vi "Generate Cartesian Trajectory.vi"   [LabVIEW 2017, in "NI_Kinematics.lvlib"]
doc: "Generates a smooth trajectory of end effector positions between two points in Cartesian space. Wire data to the <B>intermediate points</B> input to determine the polymorphic instance to use or manually select the instance.\n\n<B>.m file:</B> ctraj"
uses:
  <vilib>/robotics/Kinematics/NI_Kinematics.lvlib
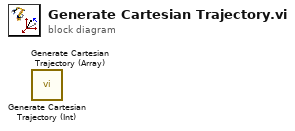
[diagram p0: block diagram]
diagram:
  n1 = call <vilib>:"Generate Cartesian Trajectory (Int).vi"() -> ()  [unwired: 10 in, 2 out]
  n2 = call <vilib>:"Generate Cartesian Trajectory (Array).vi"() -> ()  [unwired: 10 in, 2 out]
